vi "From Step Ref.vi"(8 "error in (no error)":errorcluster, 11 "Ref":refnum<k7>) -> (0 "error out":errorcluster, 3 "Step out":refnum<class "Step.lvclass">)   [LabVIEW 2020, in "TSnax.lvlib" / "Step.lvclass"]
uses:
  Step.lvclass
  Step.lvclass/Step.ctl
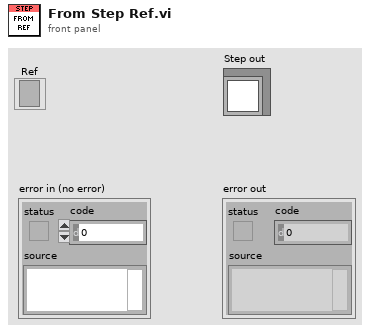
[diagram p1: front panel]
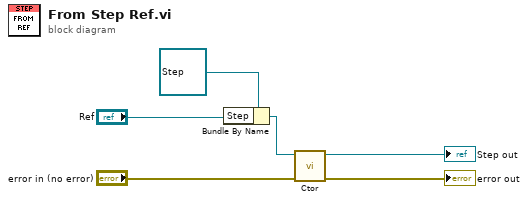
[diagram p0: block diagram]
diagram:
  n1 = Bundle By Name(cluster=refnum<class "Step.lvclass"> refnum ("Step in"), "Step"="Ref") -> (w4:refnum<class "Step.lvclass">)
  n2 = call-dynamic "Ctor.vi"("error in (no error)"="error in (no error)", "Step in"=w4) -> ("error out"=→"error out":errorcluster, "Step out"=→"Step out":refnum<class "Step.lvclass">)  [unwired: 8 in]
